vi "initalize(SubVI).vi"(4 "参考信号 1":T2, 5 "参考信号2":T2, 6 "仪器设置":T4, 7 "参考信号 3":T2, 9 "输入信号":T1, 10 "滤波设置":T3, 11 "参考信号 4":T2) -> (2 "错误输出":errorcluster)   [LabVIEW 2019, in "old.lvlib"]
uses:
  lib/Stanford Research 830/Public/Data/Read (All Parameters).vi
  old.lvlib
  lib/Stanford Research 830/Stanford Research 830.lvlib
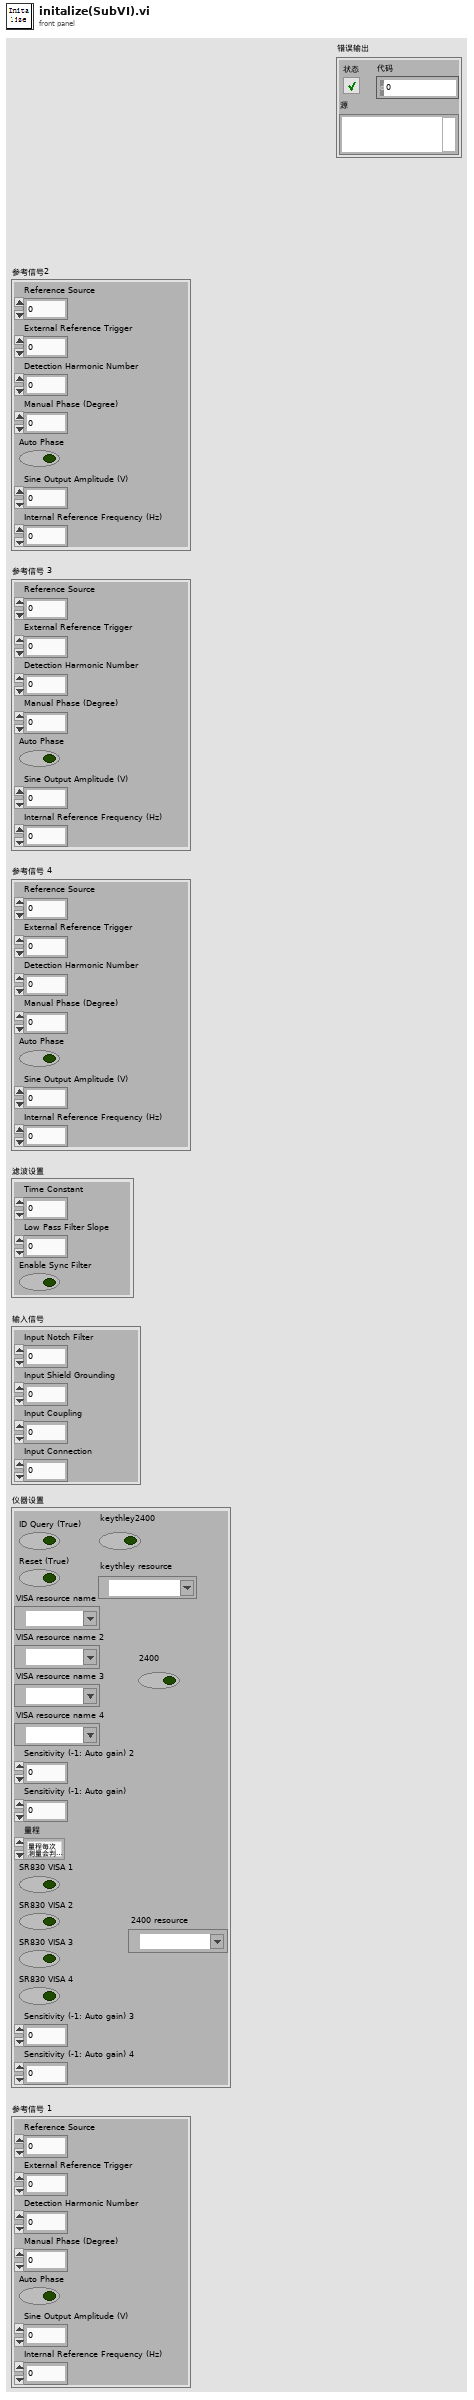
[diagram p1: front panel]
types:
  T1 = cluster{"Input Notch Filter ":u16, "Input Shield Grounding":u16, "Input Coupling ":u16, "Input Connection  ":u16}
  T2 = cluster{"Reference Source":u16, "External Reference Trigger  ":u16, "Detection Harmonic Number ":dbl, "Manual Phase (Degree)":dbl, "Auto Phase ":bool, "Sine Output Amplitude (V)":dbl, "Internal Reference Frequency (Hz)":dbl}
  T3 = cluster{"Time Constant ":u16, "Low Pass Filter Slope ":u16, "Enable Sync Filter ":bool}
  T4 = cluster{"ID Query (True)":bool, "Reset (True)":bool, "VISA resource name":refnum<visa-resource-name>, "VISA resource name 2":refnum<visa-resource-name>, "VISA resource name 3":refnum<visa-resource-name>, "VISA resource name 4":refnum<visa-resource-name>, "Sensitivity (-1: Auto gain) 2":i16, "Sensitivity (-1: Auto gain)":i16, "量程":enum16{"量程每次测量会判定", "量程不变为设定值"}, "SR830 VISA 1":bool, "SR830 VISA 2":bool, "SR830 VISA 3":bool, "SR830 VISA 4":bool, "Sensitivity (-1: Auto gain) 3":i16, "Sensitivity (-1: Auto gain) 4":i16, "keythley2400":bool, "keythley resource":refnum<visa-resource-name>, "2400":bool, "2400 resource":refnum<visa-resource-name>}
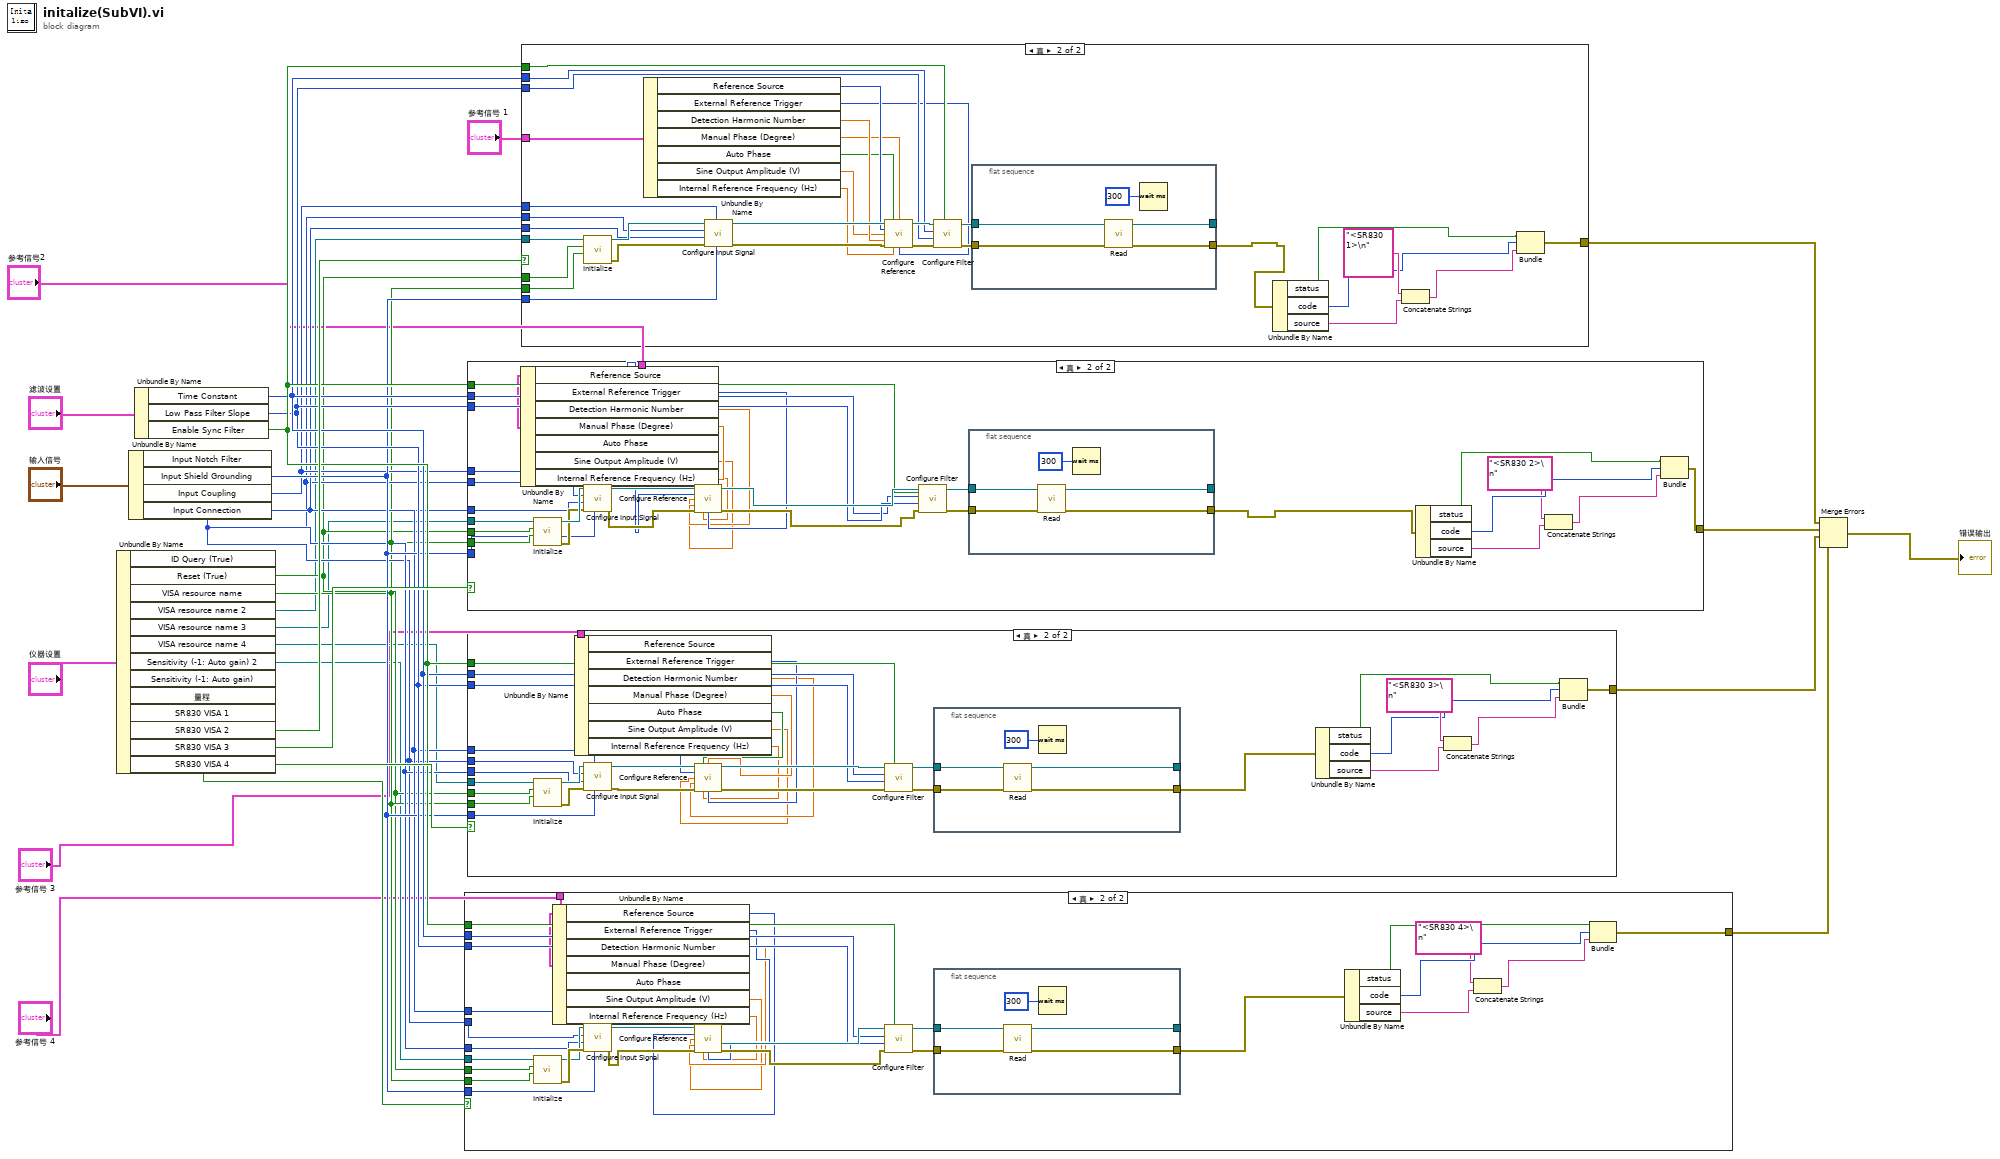
[diagram p0: block diagram]
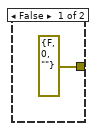
[diagram p2: hidden frame]
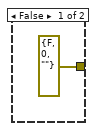
[diagram p3: hidden frame]
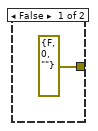
[diagram p4: hidden frame]
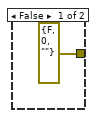
[diagram p5: hidden frame]
diagram:
  n1 = Unbundle By Name("仪器设置") -> ("ID Query (True)"=w17:bool, "Reset (True)"=w18:bool, "VISA resource name"=w11:refnum<visa-resource-name>, "VISA resource name 2"=w10:refnum<visa-resource-name>, "VISA resource name 3"=w15:refnum<visa-resource-name>, "VISA resource name 4"=w16:refnum<visa-resource-name>, "SR830 VISA 1"=w29:bool, "SR830 VISA 2"=w28:bool, "SR830 VISA 3"=w27:bool, "SR830 VISA 4"=w26:bool)  [unwired: 3 out]
  n2 = Unbundle By Name("输入信号") -> ("Input Notch Filter"=w22:u16, "Input Shield Grounding"=w21:u16, "Input Coupling"=w20:u16, "Input Connection"=w19:u16)
  n3 = Unbundle By Name("滤波设置") -> ("Time Constant"=w24:u16, "Low Pass Filter Slope"=w23:u16, "Enable Sync Filter"=w25:bool)
  n4 = case shown="真" w26 {
    tunnel: w16 -> [_ w55]
    tunnel: w17 -> [_ w54]
    tunnel: w18 -> [_ w53]
    tunnel: w19 -> [_ w52]
    tunnel: w20 -> [_ w51]
    tunnel: w21 -> [_ w50]
    tunnel: w22 -> [_ w49]
    tunnel: w23 -> [_ w48]
    tunnel: w24 -> [_ w47]
    tunnel: w25 -> [_ w46]
    tunnel: "参考信号 4" -> [_ w45]
    tunnel: [cluster{"status":bool, "code":i32, string} {"status"=FALSE, "code"=0, ""} w32] -> w2
    frame False {
    }
    frame True {
      n5 = call "Initialize.vi"("Reset (True)"=w53, "ID Query (True)"=w54, "VISA resource name"=w55) -> ("error out"=w57:errorcluster, "VISA resource name out"=w56:refnum<visa-resource-name>)  [unwired: 7 in]
      n6 = Unbundle By Name(w45) -> ("Reference Source"=w44:u16, "External Reference Trigger"=w43:u16, "Detection Harmonic Number"=w42:dbl, "Manual Phase (Degree)"=w41:dbl, "Auto Phase"=w40:bool, "Sine Output Amplitude (V)"=w39:dbl, "Internal Reference Frequency (Hz)"=w38:dbl)
      n7 = call "Configure Input Signal.vi"("Input Notch Filter (0: None)"=w49, "Input Shield Grounding (0: Float)"=w50, "error in (no error)"=w57, "Input Coupling (0: AC)"=w51, "Input Connection (0: Single-Ended Voltage)"=w52, "VISA resource name"=w56) -> ("error out"=w59:errorcluster, "VISA resource name out"=w58:refnum<visa-resource-name>)  [unwired: 4 in]
      n8 = call "Configure Reference.vi"("VISA resource name"=w58, "Auto Phase (T: Enabled)"=w40, "Manual Phase (0 Degree)"=w41, "Reference Source (1: Internal)"=w44, "Sine Output Amplitude (1 V)"=w39, "Detection Harmonic Number (1)"=w42, "error in (no error)"=w59, "Internal Reference Frequency (1000 Hz)"=w38, "External Reference Trigger (0: Sine Zero Crossing)"=w43) -> ("VISA resource name out"=w60:refnum<visa-resource-name>, "error out"=w61:errorcluster)  [unwired: 5 in]
      n9 = call "Configure Filter.vi"("Enable Sync Filter (F: Disable)"=w46, "error in (no error)"=w61, "Low Pass Filter Slope (1: 12dB/oct)"=w48, "Time Constant (8: 100ms)"=w47, "VISA resource name"=w60) -> ("error out"=w63:errorcluster, "VISA resource name out"=w62:refnum<visa-resource-name>)  [unwired: 5 in]
      n10 = flat-sequence {
        tunnel: [w68] -> w31
        tunnel: w63 -> [w67]
        tunnel: w62 -> [w66]
        tunnel: [w65] -> _
        frame #0 {
          n11 = call-poly "Read.vi"("error in (no error)"=w67, "VISA resource name"=w66) -> ("error out"=w68:errorcluster, "VISA resource name out"=w65:refnum<visa-resource-name>)  [unwired: 7 in, 1 out]
          n12 = Wait (ms)(milliseconds to wait=u32 300 ("等待时间（毫秒）")) -> ()  [unwired: 1 out]
        }
      }
      n13 = Unbundle By Name(w31) -> ("status"=w35:bool, "code"=w36:i32, "source"=w34:string)
      n14 = Concatenate Strings("<SR830 4>\n", w34) -> (w37:string)
      n15 = Bundle("status"=w35, "code"=w36, w37) -> (w32:cluster{"status":bool, "code":i32, string})  [unwired: 1 in]
    }
  }
  n16 = case shown="真" w28 {
    tunnel: w10 -> [_ w102]
    tunnel: w17 -> [_ w93]
    tunnel: w18 -> [_ w92]
    tunnel: w19 -> [_ w91]
    tunnel: w20 -> [_ w90]
    tunnel: w21 -> [_ w89]
    tunnel: w22 -> [_ w88]
    tunnel: w23 -> [_ w87]
    tunnel: w24 -> [_ w86]
    tunnel: w25 -> [_ w85]
    tunnel: "参考信号2" -> [_ w84]
    tunnel: [cluster{"status":bool, "code":i32, string} {"status"=FALSE, "code"=0, ""} w71] -> w4
    frame False {
    }
    frame True {
      n17 = Unbundle By Name(w84) -> ("Reference Source"=w83:u16, "External Reference Trigger"=w82:u16, "Detection Harmonic Number"=w81:dbl, "Manual Phase (Degree)"=w80:dbl, "Auto Phase"=w79:bool, "Sine Output Amplitude (V)"=w78:dbl, "Internal Reference Frequency (Hz)"=w77:dbl)
      n18 = call "Initialize.vi"("Reset (True)"=w92, "ID Query (True)"=w93, "VISA resource name"=w102) -> ("error out"=w100:errorcluster, "VISA resource name out"=w101:refnum<visa-resource-name>)  [unwired: 7 in]
      n19 = call "Configure Input Signal.vi"("Input Notch Filter (0: None)"=w88, "Input Shield Grounding (0: Float)"=w89, "error in (no error)"=w100, "Input Coupling (0: AC)"=w90, "Input Connection (0: Single-Ended Voltage)"=w91, "VISA resource name"=w101) -> ("error out"=w98:errorcluster, "VISA resource name out"=w99:refnum<visa-resource-name>)  [unwired: 4 in]
      n20 = call "Configure Reference.vi"("VISA resource name"=w99, "Auto Phase (T: Enabled)"=w79, "Manual Phase (0 Degree)"=w80, "Reference Source (1: Internal)"=w83, "Sine Output Amplitude (1 V)"=w78, "Detection Harmonic Number (1)"=w81, "error in (no error)"=w98, "Internal Reference Frequency (1000 Hz)"=w77, "External Reference Trigger (0: Sine Zero Crossing)"=w82) -> ("VISA resource name out"=w97:refnum<visa-resource-name>, "error out"=w96:errorcluster)  [unwired: 5 in]
      n21 = call "Configure Filter.vi"("Enable Sync Filter (F: Disable)"=w85, "error in (no error)"=w96, "Low Pass Filter Slope (1: 12dB/oct)"=w87, "Time Constant (8: 100ms)"=w86, "VISA resource name"=w97) -> ("error out"=w94:errorcluster, "VISA resource name out"=w95:refnum<visa-resource-name>)  [unwired: 5 in]
      n22 = flat-sequence {
        tunnel: [w107] -> _
        tunnel: w95 -> [w106]
        tunnel: w94 -> [w105]
        tunnel: [w104] -> w70
        frame #0 {
          n23 = call-poly "Read.vi"("error in (no error)"=w105, "VISA resource name"=w106) -> ("error out"=w104:errorcluster, "VISA resource name out"=w107:refnum<visa-resource-name>)  [unwired: 7 in, 1 out]
          n24 = Wait (ms)(milliseconds to wait=u32 300 ("等待时间（毫秒）")) -> ()  [unwired: 1 out]
        }
      }
      n25 = Unbundle By Name(w70) -> ("status"=w74:bool, "code"=w75:i32, "source"=w73:string)
      n26 = Concatenate Strings("<SR830 2>\n", w73) -> (w76:string)
      n27 = Bundle("status"=w74, "code"=w75, w76) -> (w71:cluster{"status":bool, "code":i32, string})  [unwired: 1 in]
    }
  }
  n28 = case shown="真" w27 {
    tunnel: w15 -> [_ w133]
    tunnel: w17 -> [_ w132]
    tunnel: w18 -> [_ w131]
    tunnel: w19 -> [_ w130]
    tunnel: w20 -> [_ w129]
    tunnel: w21 -> [_ w128]
    tunnel: w22 -> [_ w127]
    tunnel: w23 -> [_ w126]
    tunnel: w24 -> [_ w125]
    tunnel: w25 -> [_ w124]
    tunnel: "参考信号 3" -> [_ w123]
    tunnel: [cluster{"status":bool, "code":i32, string} {"status"=FALSE, "code"=0, ""} w110] -> w3
    frame False {
    }
    frame True {
      n29 = call "Initialize.vi"("Reset (True)"=w131, "ID Query (True)"=w132, "VISA resource name"=w133) -> ("error out"=w135:errorcluster, "VISA resource name out"=w134:refnum<visa-resource-name>)  [unwired: 7 in]
      n30 = Unbundle By Name(w123) -> ("Reference Source"=w122:u16, "External Reference Trigger"=w121:u16, "Detection Harmonic Number"=w120:dbl, "Manual Phase (Degree)"=w119:dbl, "Auto Phase"=w118:bool, "Sine Output Amplitude (V)"=w117:dbl, "Internal Reference Frequency (Hz)"=w116:dbl)
      n31 = call "Configure Input Signal.vi"("Input Notch Filter (0: None)"=w127, "Input Shield Grounding (0: Float)"=w128, "error in (no error)"=w135, "Input Coupling (0: AC)"=w129, "Input Connection (0: Single-Ended Voltage)"=w130, "VISA resource name"=w134) -> ("error out"=w137:errorcluster, "VISA resource name out"=w136:refnum<visa-resource-name>)  [unwired: 4 in]
      n32 = call "Configure Reference.vi"("VISA resource name"=w136, "Auto Phase (T: Enabled)"=w118, "Manual Phase (0 Degree)"=w119, "Reference Source (1: Internal)"=w122, "Sine Output Amplitude (1 V)"=w117, "Detection Harmonic Number (1)"=w120, "error in (no error)"=w137, "Internal Reference Frequency (1000 Hz)"=w116, "External Reference Trigger (0: Sine Zero Crossing)"=w121) -> ("VISA resource name out"=w138:refnum<visa-resource-name>, "error out"=w139:errorcluster)  [unwired: 5 in]
      n33 = call "Configure Filter.vi"("Enable Sync Filter (F: Disable)"=w124, "error in (no error)"=w139, "Low Pass Filter Slope (1: 12dB/oct)"=w126, "Time Constant (8: 100ms)"=w125, "VISA resource name"=w138) -> ("error out"=w141:errorcluster, "VISA resource name out"=w140:refnum<visa-resource-name>)  [unwired: 5 in]
      n34 = flat-sequence {
        tunnel: w141 -> [w146]
        tunnel: w140 -> [w145]
        tunnel: [w144] -> w109
        tunnel: [w143] -> _
        frame #0 {
          n35 = call-poly "Read.vi"("error in (no error)"=w146, "VISA resource name"=w145) -> ("error out"=w144:errorcluster, "VISA resource name out"=w143:refnum<visa-resource-name>)  [unwired: 7 in, 1 out]
          n36 = Wait (ms)(milliseconds to wait=u32 300 ("等待时间（毫秒）")) -> ()  [unwired: 1 out]
        }
      }
      n37 = Unbundle By Name(w109) -> ("status"=w113:bool, "code"=w112:i32, "source"=w114:string)
      n38 = Concatenate Strings("<SR830 3>\n", w114) -> (w111:string)
      n39 = Bundle("status"=w113, "code"=w112, w111) -> (w110:cluster{"status":bool, "code":i32, string})  [unwired: 1 in]
    }
  }
  n40 = case shown="真" w29 {
    tunnel: w11 -> [_ w180]
    tunnel: w17 -> [_ w171]
    tunnel: w18 -> [_ w170]
    tunnel: w19 -> [_ w169]
    tunnel: w20 -> [_ w168]
    tunnel: w21 -> [_ w167]
    tunnel: w22 -> [_ w166]
    tunnel: w23 -> [_ w165]
    tunnel: w24 -> [_ w164]
    tunnel: w25 -> [_ w163]
    tunnel: "参考信号 1" -> [_ w162]
    tunnel: [cluster{"status":bool, "code":i32, string} {"status"=FALSE, "code"=0, ""} w149] -> w5
    frame False {
    }
    frame True {
      n41 = call "Initialize.vi"("Reset (True)"=w170, "ID Query (True)"=w171, "VISA resource name"=w180) -> ("error out"=w178:errorcluster, "VISA resource name out"=w179:refnum<visa-resource-name>)  [unwired: 7 in]
      n42 = Unbundle By Name(w162) -> ("Reference Source"=w161:u16, "External Reference Trigger"=w160:u16, "Detection Harmonic Number"=w159:dbl, "Manual Phase (Degree)"=w158:dbl, "Auto Phase"=w157:bool, "Sine Output Amplitude (V)"=w156:dbl, "Internal Reference Frequency (Hz)"=w155:dbl)
      n43 = call "Configure Input Signal.vi"("Input Notch Filter (0: None)"=w166, "Input Shield Grounding (0: Float)"=w167, "error in (no error)"=w178, "Input Coupling (0: AC)"=w168, "Input Connection (0: Single-Ended Voltage)"=w169, "VISA resource name"=w179) -> ("error out"=w176:errorcluster, "VISA resource name out"=w177:refnum<visa-resource-name>)  [unwired: 4 in]
      n44 = call "Configure Reference.vi"("VISA resource name"=w177, "Auto Phase (T: Enabled)"=w157, "Manual Phase (0 Degree)"=w158, "Reference Source (1: Internal)"=w161, "Sine Output Amplitude (1 V)"=w156, "Detection Harmonic Number (1)"=w159, "error in (no error)"=w176, "Internal Reference Frequency (1000 Hz)"=w155, "External Reference Trigger (0: Sine Zero Crossing)"=w160) -> ("VISA resource name out"=w175:refnum<visa-resource-name>, "error out"=w174:errorcluster)  [unwired: 5 in]
      n45 = call "Configure Filter.vi"("Enable Sync Filter (F: Disable)"=w163, "error in (no error)"=w174, "Low Pass Filter Slope (1: 12dB/oct)"=w165, "Time Constant (8: 100ms)"=w164, "VISA resource name"=w175) -> ("error out"=w172:errorcluster, "VISA resource name out"=w173:refnum<visa-resource-name>)  [unwired: 5 in]
      n46 = flat-sequence {
        tunnel: [w185] -> _
        tunnel: w173 -> [w184]
        tunnel: w172 -> [w183]
        tunnel: [w182] -> w148
        frame #0 {
          n47 = call-poly "Read.vi"("error in (no error)"=w183, "VISA resource name"=w184) -> ("error out"=w182:errorcluster, "VISA resource name out"=w185:refnum<visa-resource-name>)  [unwired: 7 in, 1 out]
          n48 = Wait (ms)(milliseconds to wait=u32 300 ("等待时间（毫秒）")) -> ()  [unwired: 1 out]
        }
      }
      n49 = Unbundle By Name(w148) -> ("status"=w152:bool, "code"=w151:i32, "source"=w153:string)
      n50 = Concatenate Strings("<SR830 1>\n", w153) -> (w150:string)
      n51 = Bundle("status"=w152, "code"=w151, w150) -> (w149:cluster{"status":bool, "code":i32, string})  [unwired: 1 in]
    }
  }
  n52 = Merge Errors(w5, w4, w3, w2) -> (→"错误输出":errorcluster)
